vi "applyGlobalDelay.vi"(8 "error in (no error)":errorcluster, 10 "globalDelay":dbl, 11 "ScriptEvent in":refnum<class "ScriptEvent.lvclass">) -> (0 "error out":errorcluster, 3 "ScriptEvent out":refnum<class "ScriptEvent.lvclass">)   [LabVIEW 2011, in "Tools.lvlib" / "Scripting.lvlib" / "ScriptEvent.lvclass"]
uses:
  ScriptEvent.lvclass
  ScriptEvent.lvclass/ScriptEvent.ctl
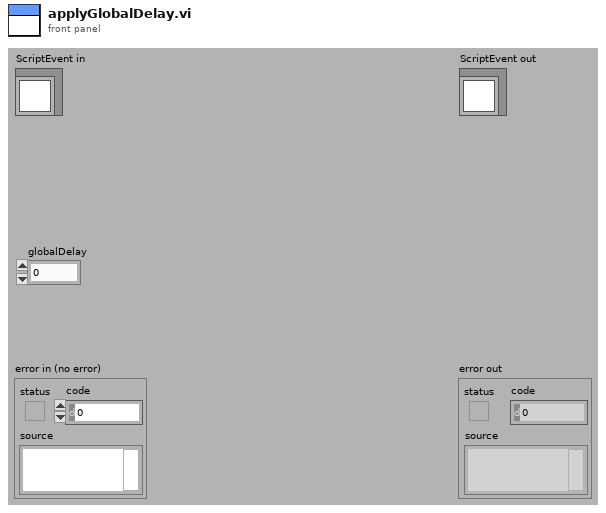
[diagram p1: front panel]
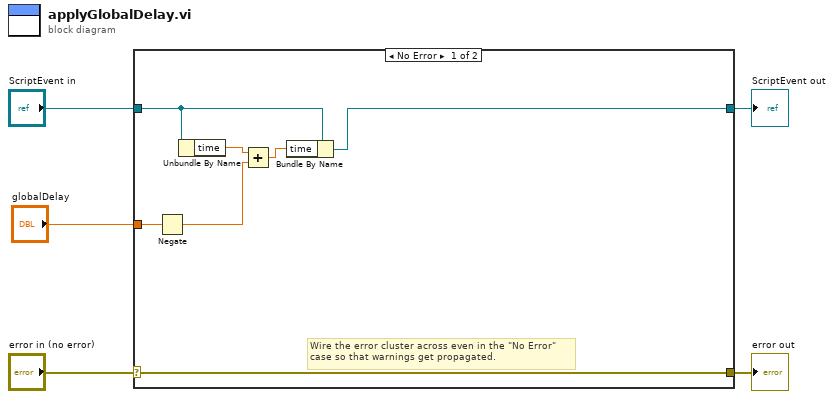
[diagram p0: block diagram]
diagram:
  n1 = case shown="No Error" "error in (no error)" {
    selector: "error in (no error)" -> [w12 w14]
    tunnel: [w12 w14] -> w4
    tunnel: [w6 w13] -> w2
    tunnel: "ScriptEvent in" -> [w7 w13]
    tunnel: "globalDelay" -> [w10 _]
    frame No Error {
      # "Wire the error cluster across even in the \"No Error\"\ncase so that warnings get propagated."
      n2 = Negate(x=w10) -> (-x=w9:dbl)
      n3 = Unbundle By Name(w7) -> ("time"=w11:dbl)
      n4 = Add(x=w11, y=w9) -> (x+y=w8:dbl)
      n5 = Bundle By Name(cluster=w7, "time"=w8) -> (w6:refnum<class "ScriptEvent.lvclass">)
    }
    frame Error {
    }
  }
  "error out" <- w4
  "ScriptEvent out" <- w2
